vi "Thev-L to Z.vi"(2 "L (mm)":dbl format="%#_13g", 3 "Frequency (Hz)":dbl[](array[numeric])) -> (0 "Zx":cdb[](array[numeric]))   [LabVIEW 2015]
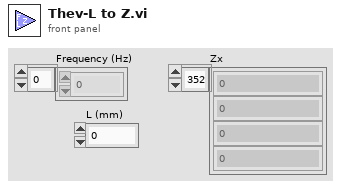
[diagram p1: front panel]
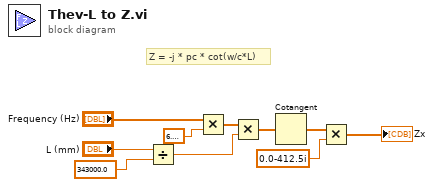
[diagram p0: block diagram]
diagram:
  # "Z = -j * pc * cot(w/c*L)"
  n1 = Divide(x="L (mm)", y=343000.0) -> (x/y=w6:dbl)
  n2 = Multiply(x="Frequency (Hz)", y=6.283185307179586) -> (x*y=w4:dbl[])
  n3 = Multiply(x=w4, y=w6) -> (x*y=w7:dbl[])
  n4 = Cotangent(1:w7) -> (0:w8:dbl[])
  n5 = Multiply(x=w8, y=cdb 0.0-412.5i) -> (x*y=→"Zx":cdb[])
